vi "SGUI Set Control Enabled State By Groups.vi"(6 "error in":errorcluster, 8 "group name to enable (none)":string) -> (7 "error out":errorcluster, 11 "enabled control references out":refnum<vi>[](array[refnum]))   [LabVIEW 2020, in "varilib.lvlib"]
doc: "This VI sets enabled states for groups of control that must be registered by calling 'SGUI Register Groups'. This VI will look for the 'group' in the stack of registered groups (registered by call of 'SGUI Register Groups'). It will start the search from last registered group and continue the search down to first registered group in the stack. If the group is found, it will enable all controls in the group and disable all controls in all other groups at the current level of stack.\n\nNote the group identifiers must be unique if you want to use the group control simultaneously in several panels!\n\nThi VI ignores input errors (will execute anyway) however will generate error if the group is not found."
uses:
  varilib.lvlib
  SGUI Global Var.vi
  <vilib>/ErrorRing/Error Ring.xnode
  <vilib>/Utility/error.llb/Error Cluster From Error Code.vi
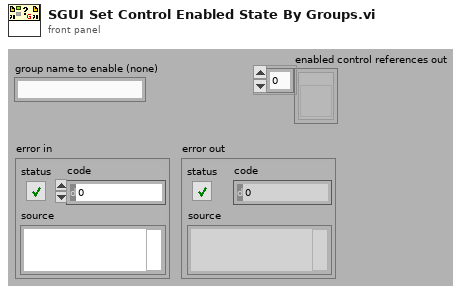
[diagram p1: front panel]
types:
  T1 = cluster{"group names":string[], "controls per goups":cluster{"control references (empty)":refnum<vi>[]}[], "ID":string}[]
  T2 = cluster{"control references (empty)":refnum<vi>[]}[]
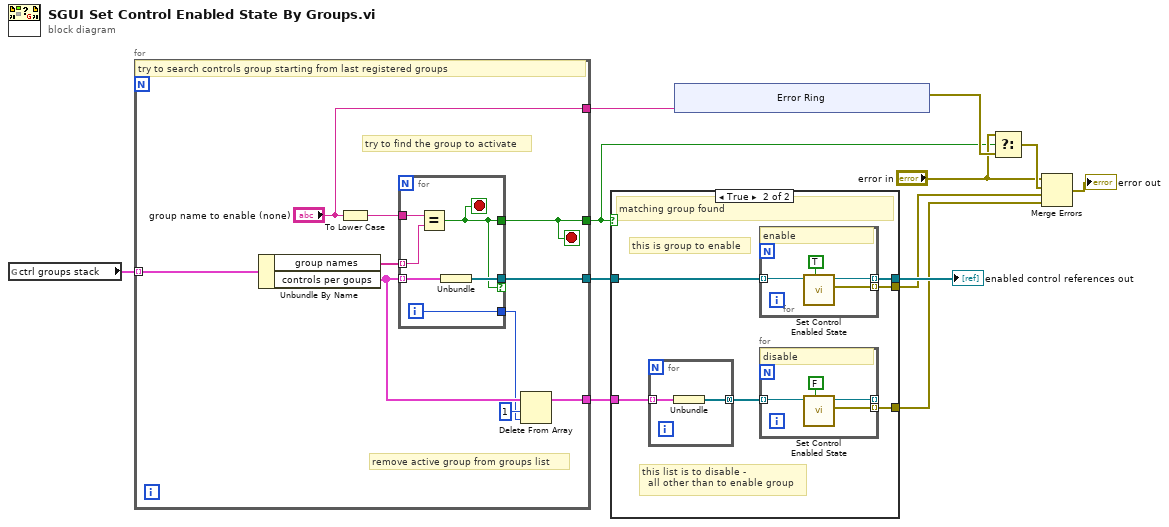
[diagram p0: block diagram]
diagram:
  n1 = global read "SGUI Global Var.vi" "ctrl groups stack"() -> (w10:T1)
  n2 = for {
    tunnel: w10 -> [w14] mode=indexing
    tunnel: [w17] -> w9
    tunnel: [w16] -> w8
    tunnel: [w13] -> w1
    tunnel: ["group name to enable (none)"] -> w5
    stop <- w13 stop-if-true
    # "remove active group from groups list"
    # "try to find the group to activate"
    # "try to search controls group starting from last registered groups"
    n3 = Unbundle By Name(w14) -> ("group names"=w21:string[], "controls per goups"=w20:T2)
    n4 = To Lower Case(string="group name to enable (none)") -> (all lower case string=w22:string)
    n5 = for {
      tunnel: w22 -> [w28]
      tunnel: w21 -> [w27] mode=indexing
      tunnel: w20 -> [w26] mode=indexing
      tunnel: [w25] -> w17 if=w23
      tunnel: [w24] -> w18
      tunnel: [w23] -> w13
      i -> [w24]
      stop <- w23 stop-if-true
      n6 = Equal?(x=w28, y=w27) -> (x = y?=w23:bool)
      n7 = Unbundle(w26) -> ("control references (empty)"=w25:refnum<vi>[])
    }
    n8 = Delete From Array(array=w20, length=1, index=w18) -> (array with subset deleted=w16:T2)  [unwired: 1 out]
  }
  n9 = case shown="True" w1 {
    tunnel: [w29 w35] -> w12
    tunnel: w9 -> [w29 w34]
    tunnel: w8 -> [_ w33]
    tunnel: [_ w31] -> w3
    tunnel: [_ w30] -> w2
    frame False {
      # "no match found!"
    }
    frame True {
      # "this list is to disable - \n  all other than to enable group"
      # "this is group to enable"
      # "matching group found"
      n10 = for {
        tunnel: w33 -> [w41] mode=indexing
        tunnel: [w40] -> w32 mode=concatenating
        n11 = Unbundle(w41) -> ("control references (empty)"=w40:refnum<vi>[])
      }
      n12 = for {
        tunnel: [w42] -> w35 mode=indexing
        tunnel: [w45] -> w31 mode=indexing
        tunnel: w34 -> [w43] mode=indexing
        # "enable"
        n13 = call "Set Control Enabled State.vi"("enabled (T)"=TRUE, "reference in"=w43) -> ("error out"=w45:errorcluster, "reference out"=w42:refnum<vi>)  [unwired: 8 in]
      }
      n14 = for {
        tunnel: [w36] -> _ mode=indexing
        tunnel: [w39] -> w30 mode=indexing
        tunnel: w32 -> [w37] mode=indexing
        # "disable"
        n15 = call "Set Control Enabled State.vi"("enabled (T)"=FALSE, "reference in"=w37) -> ("error out"=w39:errorcluster, "reference out"=w36:refnum<vi>)  [unwired: 8 in]
      }
    }
  }
  "enabled control references out" <- w12
  n16 = xnode "Error Ring"("parameter 0"=w5) -> ("error out"=w6:errorcluster)
  n17 = Select(t="error in", s=w1, f=w6) -> (s? t:f=w7:errorcluster)
  n18 = Merge Errors("error in", w7, w3, w2) -> (→"error out":errorcluster)
